vi "counter 2.vi"() -> (0 "Sum Counter 1+2":i32 caption="Gesamtanzahl", 1 "FGV value":u32 caption="Gesamtanzahl", 2 "Counter 2":i32 caption="Zählwert 1")   [LabVIEW 2023]
uses:
  cntrls/control_enum.ctl
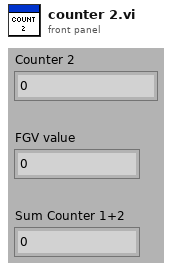
[diagram p1: front panel]
types:
  T1 = typedef "control_enum.ctl" = enum16{"read", "write", "clear"}
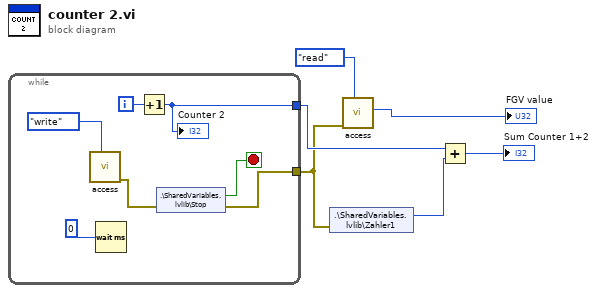
[diagram p0: block diagram]
diagram:
  n1 = while {
    tunnel: [w9] -> w5
    tunnel: [w13] -> w3
    i -> [w10]
    stop <- w11 stop-if-true
    n2 = call "access.vi"("Control_enum"=control_enum."write") -> ("error out"=w7:errorcluster)  [unwired: 7 in, 1 out]
    n3 = Wait (ms)(milliseconds to wait=u32 0) -> ()  [unwired: 1 out]
    n4 = Increment(x=w10) -> (x+1=w9:i32)
    "Counter 2" <- w9
    n5 = shared-variable ".\\SharedVariables.lvlib\\Stop"(error in=w7) -> (w11:bool, error out=w13:errorcluster)
  }
  n6 = shared-variable ".\\SharedVariables.lvlib\\Zahler1"(error in=w3) -> (w6:i32)  [unwired: 1 out]
  n7 = call "access.vi"("Control_enum"=control_enum."read", "error in (no error)"=w3) -> ("Numeric"=→"FGV value":u32)  [unwired: 6 in, 1 out]
  n8 = Add(x=w5, y=w6) -> (x+y=→"Sum Counter 1+2":i32)
